vi "Set PWM Frequency.vi"(8 "error in (no error)":errorcluster, 10 "frequency (15 kHz)":u16=15000, 11 "DC Brick in":refnum<class "DC Brick.lvclass">) -> (0 "error out":errorcluster, 3 "DC Brick out":refnum<class "DC Brick.lvclass">)   [LabVIEW 2011, in "Tinkerforge.lvlib" / "DC Brick.lvclass"]
doc: "This VI sets the frequency (in Hz) of the PWM with which the motor is driven. The possible range of the frequency is 1-20000Hz. Often a high frequency is less noisy and the motor runs smoother. However, with a low frequency there are less switches and therefore fewer switching losses. Also with most motors lower frequencies enable higher torque.\n\nIf you have no idea what all this means, just ignore this function and use the default frequency, it will very likely work fine.\n\nThe default frequency is 15 kHz."
uses:
  DC Brick.lvclass
  Device/Device.lvclass
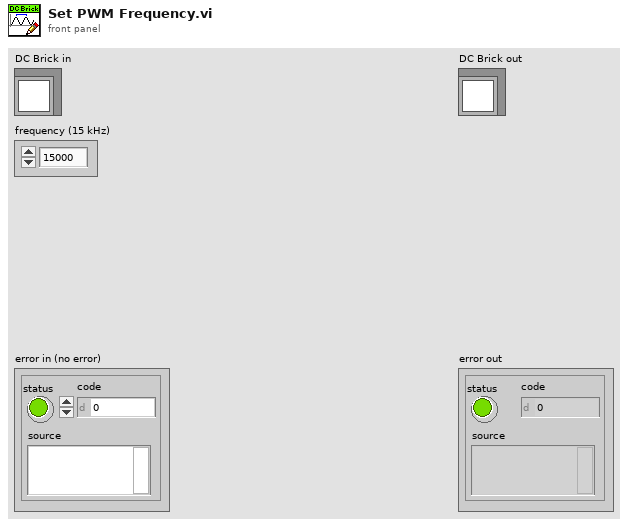
[diagram p1: front panel]
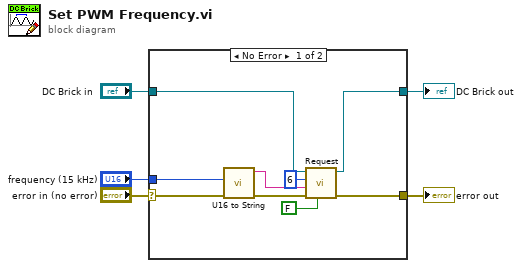
[diagram p0: block diagram]
diagram:
  n1 = case shown="No Error" "error in (no error)" {
    selector: "error in (no error)" -> [w9 w16]
    tunnel: [w10 w16] -> w4
    tunnel: [w13 w15] -> w2
    tunnel: "DC Brick in" -> [w14 w15]
    tunnel: "frequency (15 kHz)" -> [w8 _]
    frame No Error {
      n2 = call "U16 to String.vi"("Error In"=w9, "U16"=w8) -> ("Error Out"=w7:errorcluster, "String out"=w6:string)  [unwired: 8 in]
      n3 = call "Request.vi"("Response"=FALSE, "error in (no error)"=w7, "Data"=w6, "Function ID"=u8 6, "Device in"=w14) -> ("error out"=w10:errorcluster, "Device out"=w13:refnum<class "DC Brick.lvclass">)  [unwired: 2 in, 3 out]
    }
    frame Error {
    }
  }
  "error out" <- w4
  "DC Brick out" <- w2
